vi "Get Config Global Log.vi"(8 "error in (no error)":errorcluster, 11 "Global Application Log in":refnum<class "Global Application Log.lvclass">) -> (0 "error out":errorcluster, 3 "Global Application Log out":refnum<class "Global Application Log.lvclass">)   [LabVIEW 2016, in "Stream Log.lvlib" / "Global Application Log.lvclass"]
doc: "--\nCopyright © 2017 Composed SystemsI All rights reserved.\n\nAuthor: Jon McBee <jon.mcbee@composed.io>\n\nThis library is provided \"AS IS\" ,WITHOUT WARRANTIES OR\nCONDITIONS OF ANY KIND, either express or implied.\n\nComposed Systems -- composed.io\n\nStream 0.0.1.1\nJon McBee - Composed Systems\nCopyright (c) 2017, Composed Systems"
uses:
  <userlib>/Composed Systems/Stream/Log/Global Application Log/Global Application Log.lvclass
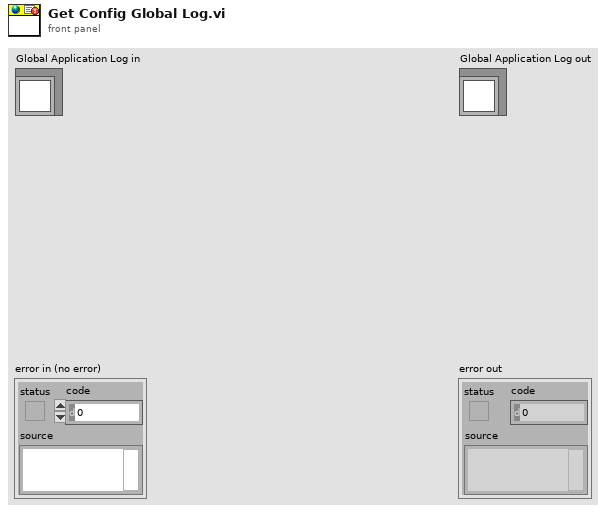
[diagram p1: front panel]
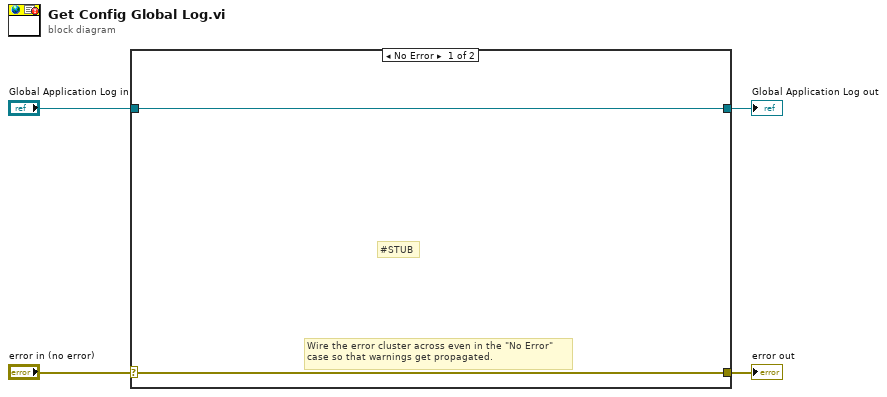
[diagram p0: block diagram]
diagram:
  n1 = case shown="No Error" "error in (no error)" {
    selector: "error in (no error)" -> [w5 w8]
    tunnel: [w5 w8] -> w3
    tunnel: [w6 w7] -> w1
    tunnel: "Global Application Log in" -> [w6 w7]
    frame No Error {
      # "#STUB"
      # "Wire the error cluster across even in the \"No Error\"\ncase so that warnings get propagated."
    }
    frame Error {
    }
  }
  "error out" <- w3
  "Global Application Log out" <- w1
